vi "Tools_String Match Wildcard Pattern String List.vi"(3 "case matching (sensitive)":T1=enum."system", 4 "pattern":string, 5 "string list":string[](array[string])=["lybraryn.llb/*", "memmon.llb/*"]) -> (0 "found pattern":bool, 1 "string":string, 2 "index":i32)   [LabVIEW 2012]
uses:
  Tools_String Case Matching.ctl
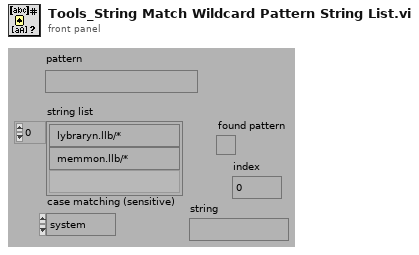
[diagram p1: front panel]
types:
  T1 = typedef "Tools_String Case Matching.ctl" = enum16{"a != A", "a == A", "system"}
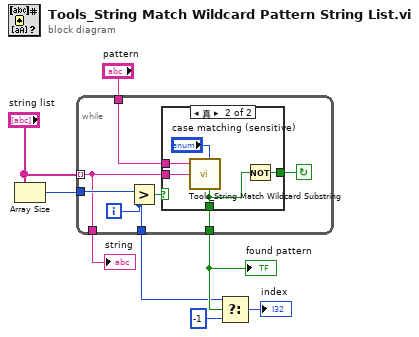
[diagram p0: block diagram]
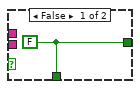
[diagram p2: hidden frame]
diagram:
  n1 = Array Size(array="string list") -> (size(s)=w6:i32)
  n2 = while {
    tunnel: [w9] -> w1
    tunnel: [w11] -> w3
    tunnel: [w13] -> w5
    tunnel: "pattern" -> [w10]
    tunnel: w6 -> [w15]
    tunnel: "string list" -> [w9] mode=indexing
    i -> [w11]
    stop <- w12 continue-if-true
    n3 = Greater?(x=w15, y=w11) -> (0:w14:bool)
    n4 = case shown="真" w14 {
      tunnel: w9 -> [_ w18]
      tunnel: [w16 w21] -> w13
      tunnel: [w16 w20] -> w12
      tunnel: w10 -> [_ w17]
      frame False {
        w16 = FALSE
      }
      frame True {
        n5 = call "Tools_String Match Wildcard Substring.vi"("case matching (sensitive)"="case matching (sensitive)", "string"=w18, "pattern with wildcards"=w17) -> ("found substring"=w21:bool)  [unwired: 1 in, 4 out]
        n6 = Not(x=w21) -> (.not. x?=w20:bool)
      }
    }
  }
  "found pattern" <- w5
  "string" <- w1
  n7 = Select(t=w3, s=w5, f=-1) -> (s? t:f=→"index":i32)
